vi "VAT_valve_get_status.vi"(8 "error in (no error)":errorcluster, 11 "VAT Valve COM port":refnum<visa-resource-name>) -> (0 "error out":errorcluster, 3 "VAT Valve COM port out":refnum<visa-resource-name>, 4 "Temperature":dbl, 5 "Version":dbl, 6 "Status":dbl, 7 "Position":dbl)   [LabVIEW 2019]
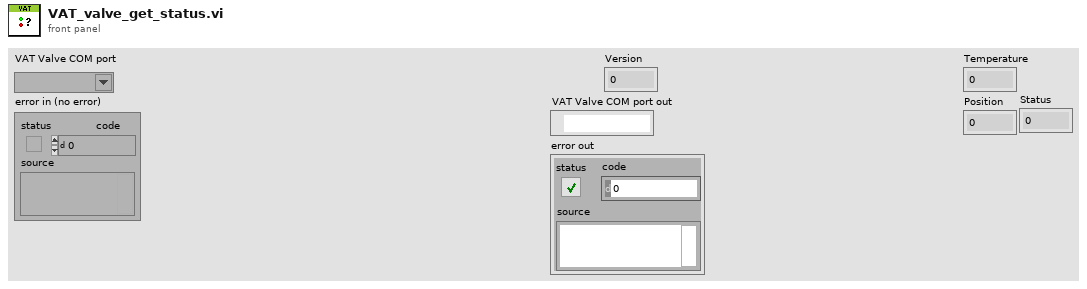
[diagram p1: front panel]
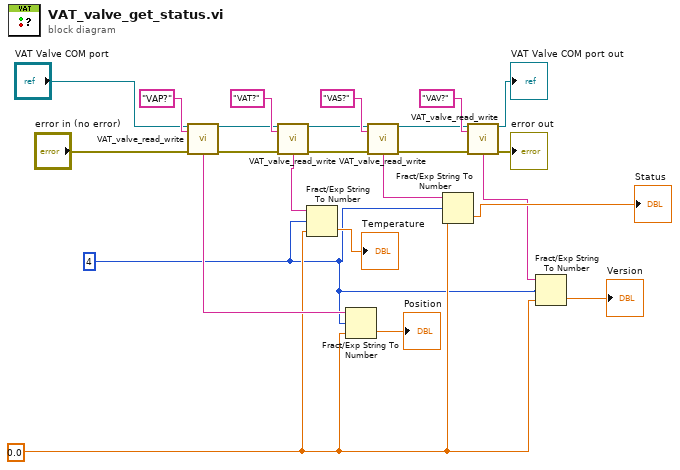
[diagram p0: block diagram]
diagram:
  w3 = 0.0
  w2 = 4 ("offset (0)")
  n1 = call "VAT_valve_read_write.vi"("VAT Valve COM port"="VAT Valve COM port", "Write String"="VAP?", "error in (no error)"="error in (no error)") -> ("VAT Valve COM port out"=w18:refnum<visa-resource-name>, "Read String"=w8:string, "error out"=w17:errorcluster)  [unwired: 10 in]
  n2 = call "VAT_valve_read_write.vi"("VAT Valve COM port"=w18, "Write String"="VAT?", "error in (no error)"=w17) -> ("VAT Valve COM port out"=w16:refnum<visa-resource-name>, "Read String"=w10:string, "error out"=w15:errorcluster)  [unwired: 10 in]
  n3 = Fract/Exp String To Number(string=w10, offset=w2, default (0 dbl)=w3) -> (number=→"Temperature":dbl)  [unwired: 1 in, 1 out]
  n4 = Fract/Exp String To Number(string=w8, offset=w2, default (0 dbl)=w3) -> (number=→"Position":dbl)  [unwired: 1 in, 1 out]
  n5 = call "VAT_valve_read_write.vi"("VAT Valve COM port"=w16, "Write String"="VAS?", "error in (no error)"=w15) -> ("VAT Valve COM port out"=w14:refnum<visa-resource-name>, "Read String"=w6:string, "error out"=w13:errorcluster)  [unwired: 10 in]
  n6 = Fract/Exp String To Number(string=w6, offset=w2, default (0 dbl)=w3) -> (number=→"Status":dbl)  [unwired: 1 in, 1 out]
  n7 = call "VAT_valve_read_write.vi"("VAT Valve COM port"=w14, "Write String"="VAV?", "error in (no error)"=w13) -> ("VAT Valve COM port out"=→"VAT Valve COM port out":refnum<visa-resource-name>, "Read String"=w4:string, "error out"=→"error out":errorcluster)  [unwired: 10 in]
  n8 = Fract/Exp String To Number(string=w4, offset=w2, default (0 dbl)=w3) -> (number=→"Version":dbl)  [unwired: 1 in, 1 out]
